vi "check should pass.vi"() -> ()   [LabVIEW 2017]
uses:
  Source/JSON Support for LabVIEW.lvlib
panel:
  out "Array":T1(array[cluster])
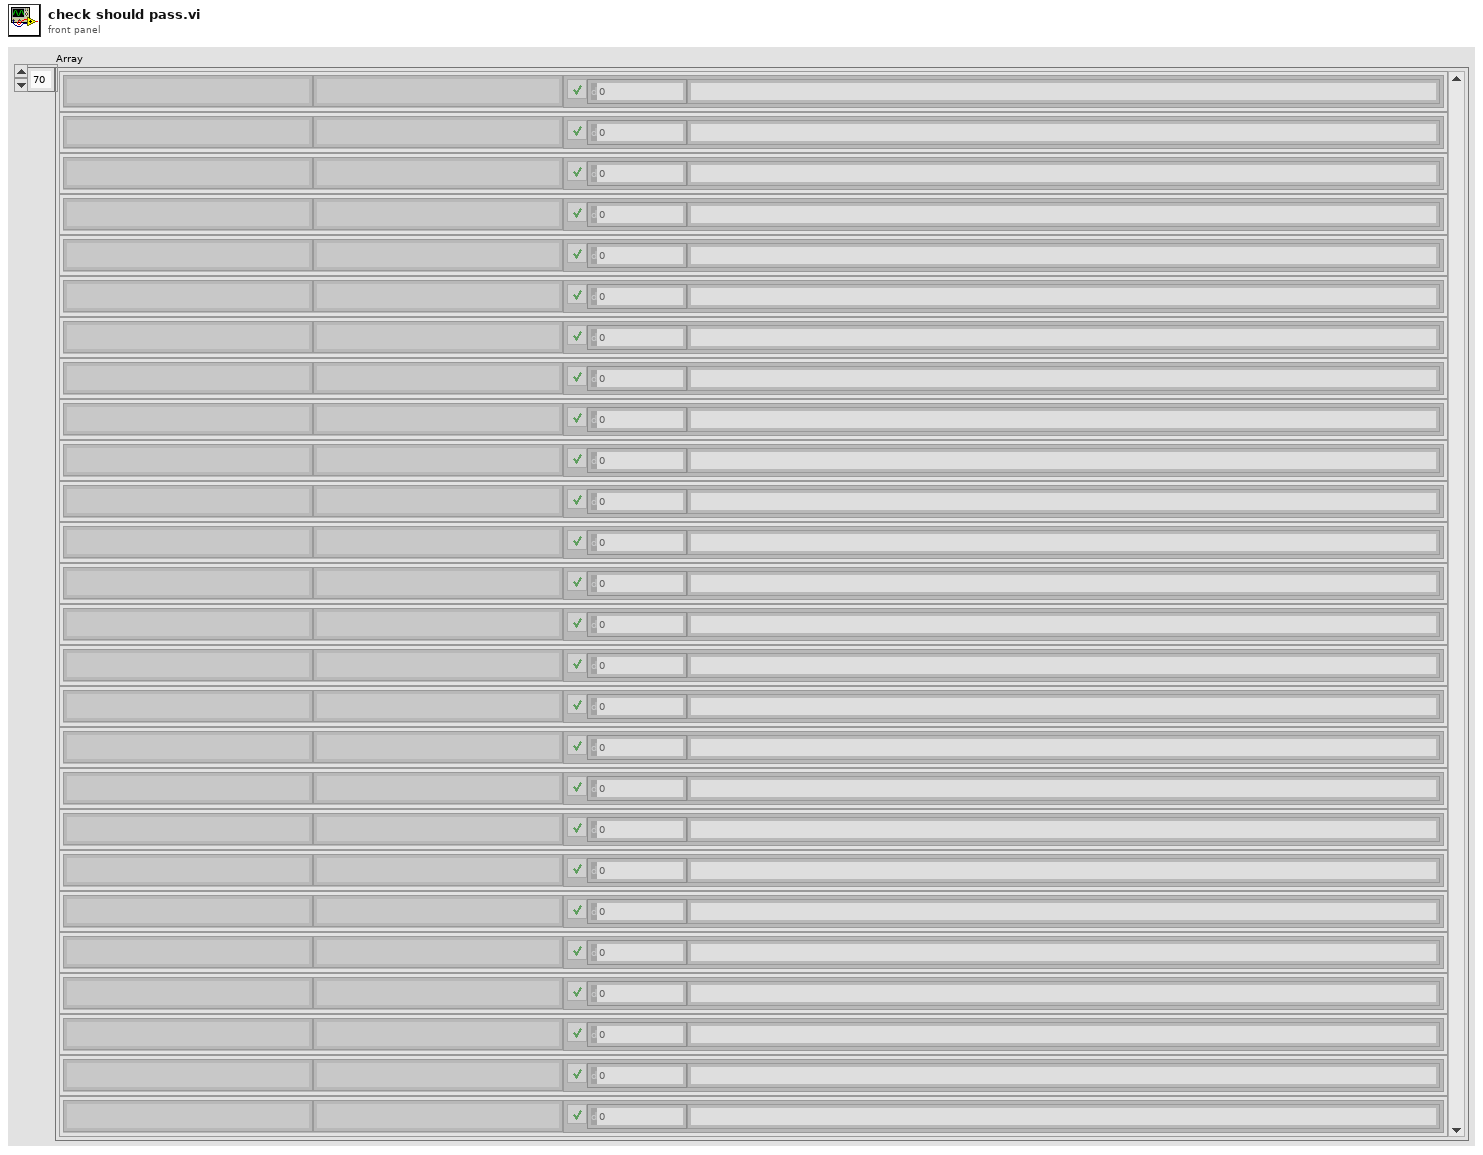
[diagram p1: front panel]
types:
  T1 = cluster{"String":string, string, "error out":errorcluster}[]
  T2 = cluster{"String":string, string, "error out":errorcluster}
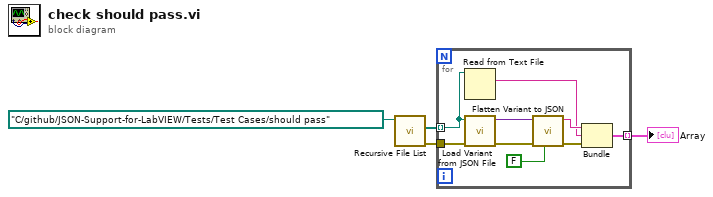
[diagram p0: block diagram]
diagram:
  n1 = call <vilib>:"Recursive File List.vi"("Folder Path"=path "C:/github/JSON-Support-for-LabVIEW/Tests/Test Cases/should pass" ("Path")) -> ("error out"=w3:errorcluster, "All Files in Dir"=w1:path[])  [unwired: 6 in, 3 out]
  n2 = for {
    tunnel: w1 -> [w10] mode=indexing
    tunnel: w3 -> [w12]
    tunnel: [w7] -> w2 mode=indexing
    n3 = Read from Text File(file (use dialog)=w10) -> (text=w8:string)  [unwired: 3 in, 3 out]
    n4 = call "Load Variant from JSON File.vi"("error in"=w12, "file path"=w10) -> ("error out"=w11:errorcluster, "JSON Value out"=w13:variant)  [unwired: 8 in]
    n5 = call "Flatten Variant to JSON.vi"("pretty print? (F)"=FALSE ("pretty print? (T)"), "error in (no error)"=w11, "JSON Value in"=w13) -> ("error out"=w6:errorcluster, "String"=w9:string)  [unwired: 7 in]
    n6 = Bundle("String"=w9, w8, "error out"=w6) -> (w7:T2)  [unwired: 1 in]
  }
  "Array" <- w2
